vi "VL6180 Init.vi"(6 "Change Slave Address":u8=255 format="%02x", 8 "Error In":errorcluster, 9 "I2C Slave Address":u8=41 format="%x", 10 "I2C Channel":u8, 11 "LINX Resource":T1) -> (0 "Error Out":errorcluster, 3 "LINX Resource":T1, 5 "VL6180 Resource":T7 {"I2C Slave Address" format="%02x"})   [LabVIEW 2014]
uses:
  <vilib>/MakerHub/LINX/Private/Type Defs/LINX Ref.ctl
  <vilib>/MakerHub/LINX/Private/Type Defs/Platform.ctl
  <vilib>/MakerHub/LINX/Private/Type Defs/Interface.ctl
  <vilib>/MakerHub/LINX/Private/Device/Type Defs/LINX Device Config.ctl
  <vilib>/MakerHub/LINX/Private/Device/Type Defs/TCP Config.ctl
  <vilib>/MakerHub/LINX/Private/Device/Type Defs/Channels.ctl
  VL6180 Resource.ctl
  VL6180X DEFS.ctl
  <vilib>/MakerHub/LINX/LMH-LINX.lvlib
  <vilib>/MakerHub/LINX/Private/Device/Device.lvlib
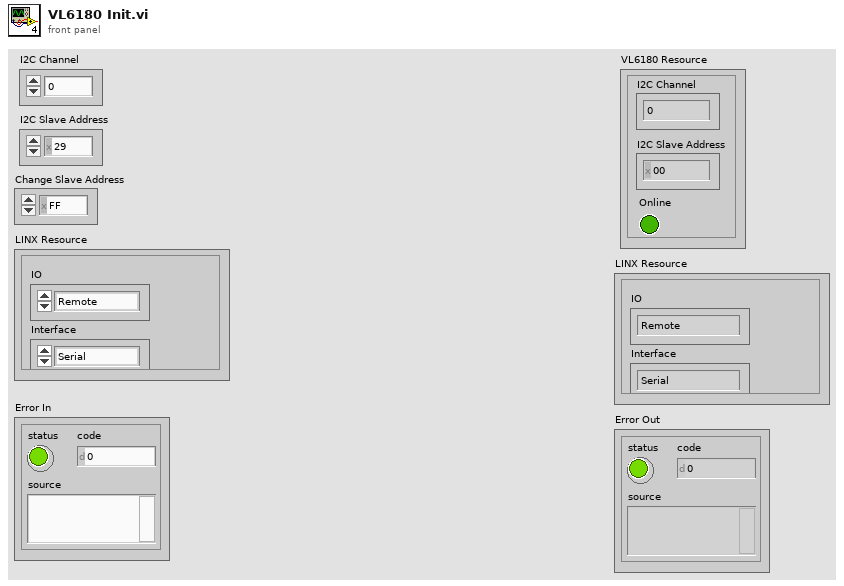
[diagram p1: front panel]
types:
  T1 = typedef "LMH-LINX.lvlib/LINX Ref.ctl" = cluster{"IO":T2, "Interface":T3, "LINX Device Config":T4}
  T2 = typedef "LMH-LINX.lvlib/Platform.ctl" = enum16{"Remote", "Local"}
  T3 = typedef "LMH-LINX.lvlib/Interface.ctl" = enum16{"Serial", "TCP"}
  T4 = typedef "LMH-LINX.lvlib/Device.lvlib/LINX Device Config.ctl" = cluster{"Interface":T3, "COM Port":refnum<visa-resource-name>, "TCP Configuration":T5, "Device Family":u8, "Device ID":u8, "Device Name":string, "TCP Ref":refnum<k5>, "Channels":T6}
  T5 = typedef "LMH-LINX.lvlib/Device.lvlib/TCP Config.ctl" = cluster{"IP Address":string, "Port":u16}
  T6 = typedef "LMH-LINX.lvlib/Channels.ctl" = cluster{"DI":u8[], "DO":u8[], "AI":u8[], "AO":u8[], "PWM":u8[], "QE":u8[], "UART":u8[], "I2C 2":u8[], "SPI":u8[], "CAN":u8[], "Servo":u8[], "AI Ref (V)":dbl, "AI Resolution (Bits)":u8, "AO Ref (V)":dbl, "AO Resolution (Bits)":u8}
  T7 = typedef "VL6180 Resource.ctl" = cluster{"I2C Channel":u8, "I2C Slave Address":u8, "Online":bool}
  T8 = typedef "VL6180X DEFS.ctl" = u16
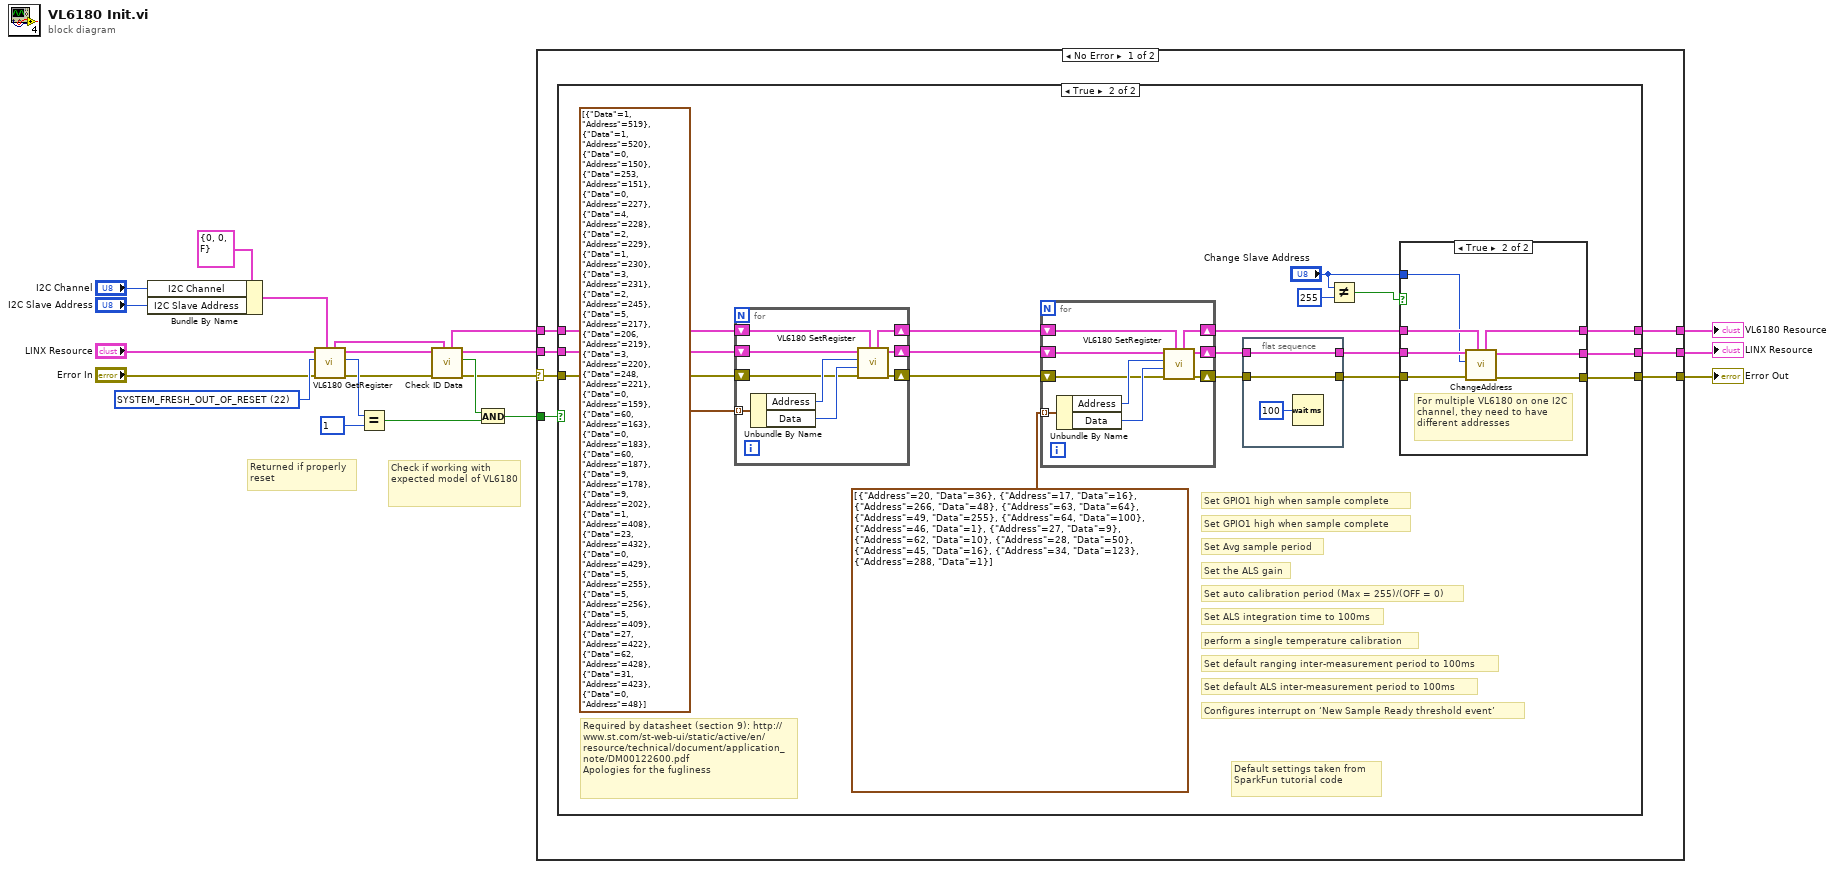
[diagram p0: block diagram]
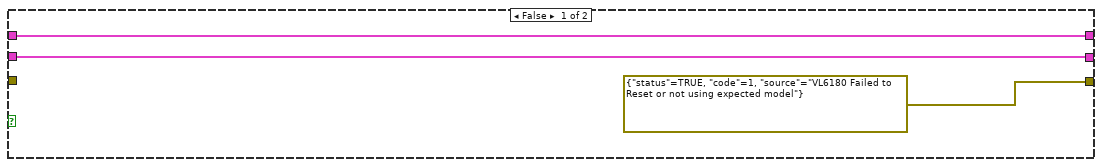
[diagram p2: hidden frame]
diagram:
  w19 = T8 22 items=["IDENTIFICATION_MODEL_ID"=0, "IDENTIFICATION_MODEL_REV_MAJOR"=1, "IDENTIFICATION_MODEL_REV_MINOR"=2, "IDENTIFICATION_MODULE_REV_MAJOR"=3, "IDENTIFICATION_MODULE_REV_MINOR"=4, "IDENTIFICATION_DATE"=6, "IDENTIFICATION_TIME"=8, "SYSTEM_MODE_GPIO0"=16, "SYSTEM_MODE_GPIO1"=17, "SYSTEM_HISTORY_CTRL"=18, "SYSTEM_INTERRUPT_CONFIG_GPIO"=20, "SYSTEM_INTERRUPT_CLEAR"=21, "SYSTEM_FRESH_OUT_OF_RESET"=22, "SYSTEM_GROUPED_PARAMETER_HOLD"=23, "SYSRANGE_START"=24, "SYSRANGE_THRESH_HIGH"=25, "SYSRANGE_THRESH_LOW"=26, "SYSRANGE_INTERMEASUREMENT_PERIOD"=27, "SYSRANGE_MAX_CONVERGENCE_TIME"=28, "SYSRANGE_CROSSTALK_COMPENSATION_RATE"=30, "SYSRANGE_CROSSTALK_VALID_HEIGHT"=33, "SYSRANGE_EARLY_CONVERGENCE_ESTIMATE"=34, "SYSRANGE_PART_TO_PART_RANGE_OFFSET"=36, "SYSRANGE_RANGE_IGNORE_VALID_HEIGHT"=37, "SYSRANGE_RANGE_IGNORE_THRESHOLD"=38, "SYSRANGE_MAX_AMBIENT_LEVEL_MULT"=44, "SYSRANGE_RANGE_CHECK_ENABLES"=45, "SYSRANGE_VHV_RECALIBRATE"=46, "SYSRANGE_VHV_REPEAT_RATE"=49, "SYSALS_START"=56, "SYSALS_THRESH_HIGH"=58, "SYSALS_THRESH_LOW"=60, "SYSALS_INTERMEASUREMENT_PERIOD"=62, "SYSALS_ANALOGUE_GAIN"=63, "SYSALS_INTEGRATION_PERIOD"=64, "RESULT_RANGE_STATUS"=77, "RESULT_ALS_STATUS"=78, "RESULT_INTERRUPT_STATUS_GPIO"=79, "RESULT_ALS_VAL"=80, "RESULT_HISTORY_BUFFER"=82, "RESULT_RANGE_VAL"=98, "RESULT_RANGE_RAW"=100, "RESULT_RANGE_RETURN_RATE"=102, "RESULT_RANGE_REFERENCE_RATE"=104, "RESULT_RANGE_RETURN_SIGNAL_COUNT"=108, "RESULT_RANGE_REFERENCE_SIGNAL_COUNT"=112, "RESULT_RANGE_RETURN_AMB_COUNT"=116, "RESULT_RANGE_REFERENCE_AMB_COUNT"=120, "RESULT_RANGE_RETURN_CONV_TIME"=124, "RESULT_RANGE_REFERENCE_CONV_TIME"=128, "READOUT_AVERAGING_SAMPLE_PERIOD"=266, "FIRMWARE_BOOTUP"=281, "FIRMWARE_RESULT_SCALER"=288, "I2C_SLAVE_DEVICE_ADDRESS"=530, "INTERLEAVED_MODE_ENABLE"=675] ("VL6180X Constants")
  # "Check if working with expected model of VL6180"
  # "Returned if properly\nreset"
  n1 = Bundle By Name(cluster=T7 {"I2C Channel"=0, "I2C Slave Address"=0, "Online"=FALSE} ("VL6180 Resource"), "I2C Channel"="I2C Channel", "I2C Slave Address"="I2C Slave Address") -> (w8:T7)
  n2 = call "VL6180 GetRegister.vi"("VL6180 Resource"=w8, "error in"="Error In", "VL6180X Constants"=w19, "LINX Resource"="LINX Resource") -> ("error out"=w14:errorcluster, "Data out"=w18:u8, "LINX Resource"=w7:T1, "VL6180 Resource"=w6:T7)  [unwired: 4 in]
  n3 = Equal?(x=w18, y=u8 1 ("Data 2")) -> (x = y?=w12:bool)
  n4 = call "Check ID Data.vi"("VL6180 Resource"=w6, "Error In"=w14, "LINX Resource"=w7) -> ("Error Out"=w9:errorcluster, "Same Model?"=w13:bool, "LINX Resource"=w15:T1, "VL6180 Resource"=w5:T7)  [unwired: 5 in]
  n5 = And(x=w13, y=w12) -> (x .and. y?=w11:bool)
  n6 = case shown="No Error" w9 {
    selector: w9 -> [w24 w83]
    tunnel: [w28 w83] -> w20
    tunnel: w15 -> [w27 w84]
    tunnel: [w26 w84] -> w4
    tunnel: w11 -> [w25 _]
    tunnel: w5 -> [w23 w82]
    tunnel: [w22 w82] -> w3
    frame No Error {
      n7 = case shown="True" w25 {
        tunnel: w24 -> [_ w48]
        tunnel: [errorcluster {"status"=TRUE, "code"=1, "source"="VL6180 Failed to Reset or not using expected model"} ("Error Out") w35] -> w28
        tunnel: w27 -> [w30 w50]
        tunnel: [w30 w36] -> w26
        tunnel: w23 -> [w29 w42]
        tunnel: [w29 w34] -> w22
        frame False {
        }
        frame True {
          # "Default settings taken from SparkFun tutorial code"
          # "Configures interrupt on ‘New Sample Ready threshold event’"
          # "Set default ALS inter-measurement period to 100ms"
          # "Set default ranging inter-measurement period to 100ms"
          # "perform a single temperature calibration"
          # "Set ALS integration time to 100ms"
          # "Set auto calibration period (Max = 255)/(OFF = 0)"
          # "Set the ALS gain"
          # "Set Avg sample period"
          # "Set GPIO1 high when sample complete"
          # "Set GPIO1 high when sample complete"
          # "Required by datasheet (section 9): http://www.st.com/st-web-ui/static/active/en/resource/technical/document/application_note/DM00122600.pdf\nApologies for the fugliness"
          n8 = for {
            tunnel: cluster{"Data":u8, "Address":u16}[] [{"Data"=1, "Address"=519}, {"Data"=1, "Address"=520}, {"Data"=0, "Address"=150}, {"Data"=253, "Address"=151}, {"Data"=0, "Address"=227}, {"Data"=4, "Address"=228}, {"Data"=2, "Address"=229}, {"Data"=1, "Address"=230}, {"Data"=3, "Address"=231}, {"Data"=2, "Address"=245}, {"Data"=5, "Address"=217}, {"Data"=206, "Address"=219}, {"Data"=3, "Address"=220}, {"Data"=248, "Address"=221}, {"Data"=0, "Address"=159}, {"Data"=60, "Address"=163}, {"Data"=0, "Address"=183}, {"Data"=60, "Address"=187}, {"Data"=9, "Address"=178}, {"Data"=9, "Address"=202}, {"Data"=1, "Address"=408}, {"Data"=23, "Address"=432}, {"Data"=0, "Address"=429}, {"Data"=5, "Address"=255}, {"Data"=5, "Address"=256}, {"Data"=5, "Address"=409}, {"Data"=27, "Address"=422}, {"Data"=62, "Address"=428}, {"Data"=31, "Address"=423}, {"Data"=0, "Address"=48}] -> [w80] mode=indexing
            shift-right: [w75] -> w45
            shift-left: w48 -> [w77]
            shift-right: [w76] -> w46
            shift-left: w50 -> [w81]
            shift-right: [w73] -> w41
            shift-left: w42 -> [w74]
            n9 = Unbundle By Name(w80) -> ("Address"=w79:u16, "Data"=w78:u8)
            n10 = call "VL6180 SetRegister.vi"("VL6180 Resource"=w74, "error in (no error)"=w77, "Data in"=w78, "Address"=w79, "LINX Resource"=w81) -> ("error out"=w75:errorcluster, "LINX Resource"=w76:T1, "VL6180 Resource"=w73:T7)  [unwired: 4 in]
          }
          n11 = for {
            tunnel: cluster{"Address":T8, "Data":u8}[] [{"Address"=20, "Data"=36}, {"Address"=17, "Data"=16}, {"Address"=266, "Data"=48}, {"Address"=63, "Data"=64}, {"Address"=49, "Data"=255}, {"Address"=64, "Data"=100}, {"Address"=46, "Data"=1}, {"Address"=27, "Data"=9}, {"Address"=62, "Data"=10}, {"Address"=28, "Data"=50}, {"Address"=45, "Data"=16}, {"Address"=34, "Data"=123}, {"Address"=288, "Data"=1}] -> [w71] mode=indexing
            shift-right: [w66] -> w43
            shift-left: w45 -> [w68]
            shift-right: [w67] -> w44
            shift-left: w46 -> [w72]
            shift-right: [w64] -> w37
            shift-left: w41 -> [w65]
            n12 = Unbundle By Name(w71) -> ("Address"=w70:T8, "Data"=w69:u8)
            n13 = call "VL6180 SetRegister.vi"("VL6180 Resource"=w65, "error in (no error)"=w68, "Data in"=w69, "Address"=w70, "LINX Resource"=w72) -> ("error out"=w66:errorcluster, "LINX Resource"=w67:T1, "VL6180 Resource"=w64:T7)  [unwired: 4 in]
          }
          n14 = flat-sequence {
            tunnel: w44 -> [w63]
            tunnel: w43 -> [w62]
            tunnel: [w63] -> w39
            tunnel: [w62] -> w38
            frame #0 {
              n15 = Wait (ms)(milliseconds to wait=u32 100) -> ()  [unwired: 1 out]
            }
          }
          n16 = Not Equal?(x="Change Slave Address", y=u8 255 ("Change Slave Address")) -> (x != y?=w33:bool)
          n17 = case shown="True" w33 {
            tunnel: w39 -> [w52 w60]
            tunnel: w38 -> [w51 w56]
            tunnel: w37 -> [w53 w59]
            tunnel: [w52 w58] -> w36
            tunnel: [w51 w57] -> w35
            tunnel: [w53 w55] -> w34
            tunnel: "Change Slave Address" -> [_ w54]
            frame False {
            }
            frame True {
              # "For multiple VL6180 on one I2C channel, they need to have different addresses"
              n18 = call "ChangeAddress.vi"("VL6180 Resource"=w59, "error in"=w56, "New Slave Address"=w54, "LINX Resource"=w60) -> ("error out"=w57:errorcluster, "LINX Resource"=w58:T1, "VL6180 Resource"=w55:T7)  [unwired: 5 in]
            }
          }
        }
      }
    }
    frame Error {
    }
  }
  "Error Out" <- w20
  "VL6180 Resource" <- w3
  "LINX Resource" <- w4
